vi "Init_Advise.vi"(0 "service":string="ROBCOMM", 1 "VARIABLE TO ADVISE OF CHANGE":string="TF") -> (2 "advise refnum":u32, 3 "Current Value":string, 4 "error out":errorcluster)   [LabVIEW 2012]
panel:
  out "Command":string="VARIABLE"
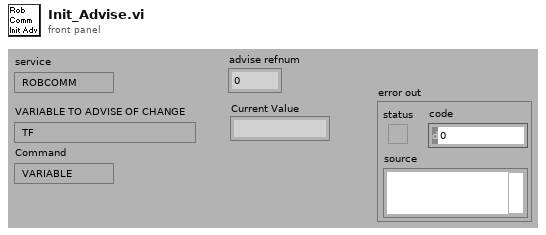
[diagram p1: front panel]
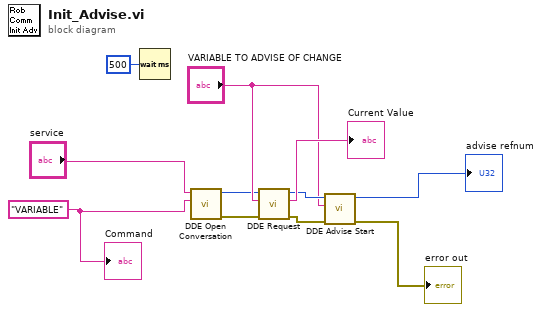
[diagram p0: block diagram]
diagram:
  w1 = "VARIABLE" ("Command")
  n1 = Wait (ms)(milliseconds to wait=u32 500) -> ()  [unwired: 1 out]
  n2 = call <vilib>:"DDE Open Conversation.vi"("topic"=w1, "service"="service") -> ("error out"=w6:errorcluster, "conversation refnum"=w7:u32)  [unwired: 6 in]
  n3 = call <vilib>:"DDE Request.vi"("error in (no error)"=w6, "item"="VARIABLE TO ADVISE OF CHANGE", "conversation refnum in"=w7) -> ("error out"=w10:errorcluster, "data"=→"Current Value":string, "conversation refnum out"=w9:u32)  [unwired: 4 in]
  n4 = call <vilib>:"DDE Advise Start.vi"("error in (no error)"=w10, "item"="VARIABLE TO ADVISE OF CHANGE", "conversation refnum"=w9) -> ("error out"=→"error out":errorcluster, "advise refnum"=→"advise refnum":u32)  [unwired: 5 in]
  "Command" <- w1
